vi "App - analyze RUS V6.vi"() -> ()   [LabVIEW 2015] (continued)
"radius"=0.0}}, "timestamp(min)"=1864.0666666701436, "timestamp"=timestamp(3493839665 s since 1904-01-01), "Magn Field(T)"=0.0}, {"temperature"=23.436, "lorentzian"={"Amplitude"=0.0, "omega(0)"=0.0, "Gamma"=0.0, "phase"=0.0, "Q"=0.0, "Norm  Ampl"=0.0, "z (inf)"=0.0+0.0i, "4corners"={"z (-pi/2)"=0.0+0.0i, "z(inf)"=0.0+0.0i, "z (pi/2)"=0.0+0.0i, "z center"=0.0+0.0i, "z(0)"=0.0+0.0i, "radius"=0.0}}, "timestamp(min)"=1865.3833333328366, "timestamp"=timestamp(3493839744 s since 1904-01-01), "Magn Field(T)"=0.0}, {"temperature"=23.334, "lorentzian"={"Amplitude"=0.0, "omega(0)"=0.0, "Gamma"=0.0, "phase"=0.0, "Q"=0.0, "Norm  Ampl"=0.0, "z (inf)"=0.0+0.0i, "4corners"={"z (-pi/2)"=0.0+0.0i, "z(inf)"=0.0+0.0i, "z (pi/2)"=0.0+0.0i, "z center"=0.0+0.0i, "z(0)"=0.0+0.0i, "radius"=0.0}}, "timestamp(min)"=1866.7000000029802, "timestamp"=timestamp(3493839823 s since 1904-01-01), "Magn Field(T)"=0.0}, {"temperature"=23.235, "lorentzian"={"Amplitude"=0.0, "omega(0)"=0.0, "Gamma"=0.0, "phase"=0.0, "Q"=0.0, "Norm  Ampl"=0.0, "z (inf)"=0.0+0.0i, "4corners"={"z (-pi/2)"=0.0+0.0i, "z(inf)"=0.0+0.0i, "z (pi/2)"=0.0+0.0i, "z center"=0.0+0.0i, "z(0)"=0.0+0.0i, "radius"=0.0}}, "timestamp(min)"=1868.0333333313465, "timestamp"=timestamp(3493839903 s since 1904-01-01), "Magn Field(T)"=0.0}, {"temperature"=23.139, "lorentzian"={"Amplitude"=0.0, "omega(0)"=0.0, "Gamma"=0.0, "phase"=0.0, "Q"=0.0, "Norm  Ampl"=0.0, "z (inf)"=0.0+0.0i, "4corners"={"z (-pi/2)"=0.0+0.0i, "z(inf)"=0.0+0.0i, "z (pi/2)"=0.0+0.0i, "z center"=0.0+0.0i, "z(0)"=0.0+0.0i, "radius"=0.0}}, "timestamp(min)"=1869.3500000014901, "timestamp"=timestamp(3493839982 s since 1904-01-01), "Magn Field(T)"=0.0}, {"temperature"=23.041, "lorentzian"={"Amplitude"=0.0, "omega(0)"=0.0, "Gamma"=0.0, "phase"=0.0, "Q"=0.0, "Norm  Ampl"=0.0, "z (inf)"=0.0+0.0i, "4corners"={"z (-pi/2)"=0.0+0.0i, "z(inf)"=0.0+0.0i, "z (pi/2)"=0.0+0.0i, "z center"=0.0+0.0i, "z(0)"=0.0+0.0i, "radius"=0.0}}, "timestamp(min)"=1870.683333337307, "timestamp"=timestamp(3493840062 s since 1904-01-01), "Magn Field(T)"=0.0}, {"temperature"=22.937, "lorentzian"={"Amplitude"=0.0, "omega(0)"=0.0, "Gamma"=0.0, "phase"=0.0, "Q"=0.0, "Norm  Ampl"=0.0, "z (inf)"=0.0+0.0i, "4corners"={"z (-pi/2)"=0.0+0.0i, "z(inf)"=0.0+0.0i, "z (pi/2)"=0.0+0.0i, "z center"=0.0+0.0i, "z(0)"=0.0+0.0i, "radius"=0.0}}, "timestamp(min)"=1872.0, "timestamp"=timestamp(3493840141 s since 1904-01-01), "Magn Field(T)"=0.0}, {"temperature"=22.842, "lorentzian"={"Amplitude"=0.0, "omega(0)"=0.0, "Gamma"=0.0, "phase"=0.0, "Q"=0.0, "Norm  Ampl"=0.0, "z (inf)"=0.0+0.0i, "4corners"={"z (-pi/2)"=0.0+0.0i, "z(inf)"=0.0+0.0i, "z (pi/2)"=0.0+0.0i, "z center"=0.0+0.0i, "z(0)"=0.0+0.0i, "radius"=0.0}}, "timestamp(min)"=1873.3166666701436, "timestamp"=timestamp(3493840220 s since 1904-01-01), "Magn Field(T)"=0.0}, {"temperature"=22.748, "lorentzian"={"Amplitude"=0.0, "omega(0)"=0.0, "Gamma"=0.0, "phase"=0.0, "Q"=0.0, "Norm  Ampl"=0.0, "z (inf)"=0.0+0.0i, "4corners"={"z (-pi/2)"=0.0+0.0i, "z(inf)"=0.0+0.0i, "z (pi/2)"=0.0+0.0i, "z center"=0.0+0.0i, "z(0)"=0.0+0.0i, "radius"=0.0}}, "timestamp(min)"=1874.6499999985099, "timestamp"=timestamp(3493840300 s since 1904-01-01), "Magn Field(T)"=0.0}, {"temperature"=22.644, "lorentzian"={"Amplitude"=0.0, "omega(0)"=0.0, "Gamma"=0.0, "phase"=0.0, "Q"=0.0, "Norm  Ampl"=0.0, "z (inf)"=0.0+0.0i, "4corners"={"z (-pi/2)"=0.0+0.0i, "z(inf)"=0.0+0.0i, "z (pi/2)"=0.0+0.0i, "z center"=0.0+0.0i, "z(0)"=0.0+0.0i, "radius"=0.0}}, "timestamp(min)"=1875.9666666686535, "timestamp"=timestamp(3493840379 s since 1904-01-01), "Magn Field(T)"=0.0}, {"temperature"=22.549, "lorentzian"={"Amplitude"=0.0, "omega(0)"=0.0, "Gamma"=0.0, "phase"=0.0, "Q"=0.0, "Norm  Ampl"=0.0, "z (inf)"=0.0+0.0i, "4corners"={"z (-pi/2)"=0.0+0.0i, "z(inf)"=0.0+0.0i, "z (pi/2)"=0.0+0.0i, "z center"=0.0+0.0i, "z(0)"=0.0+0.0i, "radius"=0.0}}, "timestamp(min)"=1877.2833333313465, "timestamp"=timestamp(3493840458 s since 1904-01-01), "Magn Field(T)"=0.0}, {"temperature"=22.448, "lorentzian"={"Amplitude"=0.0, "omega(0)"=0.0, "Gamma"=0.0, "phase"=0.0, "Q"=0.0, "Norm  Ampl"=0.0, "z (inf)"=0.0+0.0i, "4corners"={"z (-pi/2)"=0.0+0.0i, "z(inf)"=0.0+0.0i, "z (pi/2)"=0.0+0.0i, "z center"=0.0+0.0i, "z(0)"=0.0+0.0i, "radius"=0.0}}, "timestamp(min)"=1878.6166666671634, "timestamp"=timestamp(3493840538 s since 1904-01-01), "Magn Field(T)"=0.0}, {"temperature"=22.345, "lorentzian"={"Amplitude"=0.0, "omega(0)"=0.0, "Gamma"=0.0, "phase"=0.0, "Q"=0.0, "Norm  Ampl"=0.0, "z (inf)"=0.0+0.0i, "4corners"={"z (-pi/2)"=0.0+0.0i, "z(inf)"=0.0+0.0i, "z (pi/2)"=0.0+0.0i, "z center"=0.0+0.0i, "z(0)"=0.0+0.0i, "radius"=0.0}}, "timestamp(min)"=1879.933333337307, "timestamp"=timestamp(3493840617 s since 1904-01-01), "Magn Field(T)"=0.0}, {"temperature"=22.254, "lorentzian"={"Amplitude"=0.0, "omega(0)"=0.0, "Gamma"=0.0, "phase"=0.0, "Q"=0.0, "Norm  Ampl"=0.0, "z (inf)"=0.0+0.0i, "4corners"={"z (-pi/2)"=0.0+0.0i, "z(inf)"=0.0+0.0i, "z (pi/2)"=0.0+0.0i, "z center"=0.0+0.0i, "z(0)"=0.0+0.0i, "radius"=0.0}}, "timestamp(min)"=1881.2666666656733, "timestamp"=timestamp(3493840697 s since 1904-01-01), "Magn Field(T)"=0.0}, {"temperature"=22.148, "lorentzian"={"Amplitude"=0.0, "omega(0)"=0.0, "Gamma"=0.0, "phase"=0.0, "Q"=0.0, "Norm  Ampl"=0.0, "z (inf)"=0.0+0.0i, "4corners"={"z (-pi/2)"=0.0+0.0i, "z(inf)"=0.0+0.0i, "z (pi/2)"=0.0+0.0i, "z center"=0.0+0.0i, "z(0)"=0.0+0.0i, "radius"=0.0}}, "timestamp(min)"=1882.5833333358169, "timestamp"=timestamp(3493840776 s since 1904-01-01), "Magn Field(T)"=0.0}, {"temperature"=22.046, "lorentzian"={"Amplitude"=0.0, "omega(0)"=0.0, "Gamma"=0.0, "phase"=0.0, "Q"=0.0, "Norm  Ampl"=0.0, "z (inf)"=0.0+0.0i, "4corners"={"z (-pi/2)"=0.0+0.0i, "z(inf)"=0.0+0.0i, "z (pi/2)"=0.0+0.0i, "z center"=0.0+0.0i, "z(0)"=0.0+0.0i, "radius"=0.0}}, "timestamp(min)"=1883.8999999985099, "timestamp"=timestamp(3493840855 s since 1904-01-01), "Magn Field(T)"=0.0}, {"temperature"=21.957, "lorentzian"={"Amplitude"=0.0, "omega(0)"=0.0, "Gamma"=0.0, "phase"=0.0, "Q"=0.0, "Norm  Ampl"=0.0, "z (inf)"=0.0+0.0i, "4corners"={"z (-pi/2)"=0.0+0.0i, "z(inf)"=0.0+0.0i, "z (pi/2)"=0.0+0.0i, "z center"=0.0+0.0i, "z(0)"=0.0+0.0i, "radius"=0.0}}, "timestamp(min)"=1885.2333333343267, "timestamp"=timestamp(3493840935 s since 1904-01-01), "Magn Field(T)"=0.0}, {"temperature"=21.851, "lorentzian"={"Amplitude"=0.0, "omega(0)"=0.0, "Gamma"=0.0, "phase"=0.0, "Q"=0.0, "Norm  Ampl"=0.0, "z (inf)"=0.0+0.0i, "4corners"={"z (-pi/2)"=0.0+0.0i, "z(inf)"=0.0+0.0i, "z (pi/2)"=0.0+0.0i, "z center"=0.0+0.0i, "z(0)"=0.0+0.0i, "radius"=0.0}}, "timestamp(min)"=1886.5500000044703, "timestamp"=timestamp(3493841014 s since 1904-01-01), "Magn Field(T)"=0.0}, {"temperature"=21.755, "lorentzian"={"Amplitude"=0.0, "omega(0)"=0.0, "Gamma"=0.0, "phase"=0.0, "Q"=0.0, "Norm  Ampl"=0.0, "z (inf)"=0.0+0.0i, "4corners"={"z (-pi/2)"=0.0+0.0i, "z(inf)"=0.0+0.0i, "z (pi/2)"=0.0+0.0i, "z center"=0.0+0.0i, "z(0)"=0.0+0.0i, "radius"=0.0}}, "timestamp(min)"=1887.8833333328366, "timestamp"=timestamp(3493841094 s since 1904-01-01), "Magn Field(T)"=0.0}, {"temperature"=21.657, "lorentzian"={"Amplitude"=0.0, "omega(0)"=0.0, "Gamma"=0.0, "phase"=0.0, "Q"=0.0, "Norm  Ampl"=0.0, "z (inf)"=0.0+0.0i, "4corners"={"z (-pi/2)"=0.0+0.0i, "z(inf)"=0.0+0.0i, "z (pi/2)"=0.0+0.0i, "z center"=0.0+0.0i, "z(0)"=0.0+0.0i, "radius"=0.0}}, "timestamp(min)"=1889.2000000029802, "timestamp"=timestamp(3493841173 s since 1904-01-01), "Magn Field(T)"=0.0}, {"temperature"=21.553, "lorentzian"={"Amplitude"=0.0, "omega(0)"=0.0, "Gamma"=0.0, "phase"=0.0, "Q"=0.0, "Norm  Ampl"=0.0, "z (inf)"=0.0+0.0i, "4corners"={"z (-pi/2)"=0.0+0.0i, "z(inf)"=0.0+0.0i, "z (pi/2)"=0.0+0.0i, "z center"=0.0+0.0i, "z(0)"=0.0+0.0i, "radius"=0.0}}, "timestamp(min)"=1890.5166666656733, "timestamp"=timestamp(3493841252 s since 1904-01-01), "Magn Field(T)"=0.0}, {"temperature"=21.455, "lorentzian"={"Amplitude"=0.0, "omega(0)"=0.0, "Gamma"=0.0, "phase"=0.0, "Q"=0.0, "Norm  Ampl"=0.0, "z (inf)"=0.0+0.0i, "4corners"={"z (-pi/2)"=0.0+0.0i, "z(inf)"=0.0+0.0i, "z (pi/2)"=0.0+0.0i, "z center"=0.0+0.0i, "z(0)"=0.0+0.0i, "radius"=0.0}}, "timestamp(min)"=1891.8500000014901, "timestamp"=timestamp(3493841332 s since 1904-01-01), "Magn Field(T)"=0.0}, {"temperature"=21.36, "lorentzian"={"Amplitude"=0.0, "omega(0)"=0.0, "Gamma"=0.0, "phase"=0.0, "Q"=0.0, "Norm  Ampl"=0.0, "z (inf)"=0.0+0.0i, "4corners"={"z (-pi/2)"=0.0+0.0i, "z(inf)"=0.0+0.0i, "z (pi/2)"=0.0+0.0i, "z center"=0.0+0.0i, "z(0)"=0.0+0.0i, "radius"=0.0}}, "timestamp(min)"=1893.1666666641831, "timestamp"=timestamp(3493841411 s since 1904-01-01), "Magn Field(T)"=0.0}, {"temperature"=21.259, "lorentzian"={"Amplitude"=0.0, "omega(0)"=0.0, "Gamma"=0.0, "phase"=0.0, "Q"=0.0, "Norm  Ampl"=0.0, "z (inf)"=0.0+0.0i, "4corners"={"z (-pi/2)"=0.0+0.0i, "z(inf)"=0.0+0.0i, "z (pi/2)"=0.0+0.0i, "z center"=0.0+0.0i, "z(0)"=0.0+0.0i, "radius"=0.0}}, "timestamp(min)"=1894.4833333343267, "timestamp"=timestamp(3493841490 s since 1904-01-01), "Magn Field(T)"=0.0}, {"temperature"=21.158, "lorentzian"={"Amplitude"=0.0, "omega(0)"=0.0, "Gamma"=0.0, "phase"=0.0, "Q"=0.0, "Norm  Ampl"=0.0, "z (inf)"=0.0+0.0i, "4corners"={"z (-pi/2)"=0.0+0.0i, "z(inf)"=0.0+0.0i, "z (pi/2)"=0.0+0.0i, "z center"=0.0+0.0i, "z(0)"=0.0+0.0i, "radius"=0.0}}, "timestamp(min)"=1895.8166666701436, "timestamp"=timestamp(3493841570 s since 1904-01-01), "Magn Field(T)"=0.0}, {"temperature"=21.06, "lorentzian"={"Amplitude"=0.0, "omega(0)"=0.0, "Gamma"=0.0, "phase"=0.0, "Q"=0.0, "Norm  Ampl"=0.0, "z (inf)"=0.0+0.0i, "4corners"={"z (-pi/2)"=0.0+0.0i, "z(inf)"=0.0+0.0i, "z (pi/2)"=0.0+0.0i, "z center"=0.0+0.0i, "z(0)"=0.0+0.0i, "radius"=0.0}}, "timestamp(min)"=1897.1333333328366, "timestamp"=timestamp(3493841649 s since 1904-01-01), "Magn Field(T)"=0.0}, {"temperature"=20.959, "lorentzian"={"Amplitude"=0.0, "omega(0)"=0.0, "Gamma"=0.0, "phase"=0.0, "Q"=0.0, "Norm  Ampl"=0.0, "z (inf)"=0.0+0.0i, "4corners"={"z (-pi/2)"=0.0+0.0i, "z(inf)"=0.0+0.0i, "z (pi/2)"=0.0+0.0i, "z center"=0.0+0.0i, "z(0)"=0.0+0.0i, "radius"=0.0}}, "timestamp(min)"=1898.4666666686535, "timestamp"=timestamp(3493841729 s since 1904-01-01), "Magn Field(T)"=0.0}, {"temperature"=20.861, "lorentzian"={"Amplitude"=0.0, "omega(0)"=0.0, "Gamma"=0.0, "phase"=0.0, "Q"=0.0, "Norm  Ampl"=0.0, "z (inf)"=0.0+0.0i, "4corners"={"z (-pi/2)"=0.0+0.0i, "z(inf)"=0.0+0.0i, "z (pi/2)"=0.0+0.0i, "z center"=0.0+0.0i, "z(0)"=0.0+0.0i, "radius"=0.0}}, "timestamp(min)"=1899.7833333313465, "timestamp"=timestamp(3493841808 s since 1904-01-01), "Magn Field(T)"=0.0}, {"temperature"=20.758, "lorentzian"={"Amplitude"=0.0, "omega(0)"=0.0, "Gamma"=0.0, "phase"=0.0, "Q"=0.0, "Norm  Ampl"=0.0, "z (inf)"=0.0+0.0i, "4corners"={"z (-pi/2)"=0.0+0.0i, "z(inf)"=0.0+0.0i, "z (pi/2)"=0.0+0.0i, "z center"=0.0+0.0i, "z(0)"=0.0+0.0i, "radius"=0.0}}, "timestamp(min)"=1901.1000000014901, "timestamp"=timestamp(3493841887 s since 1904-01-01), "Magn Field(T)"=0.0}, {"temperature"=20.654, "lorentzian"={"Amplitude"=0.0, "omega(0)"=0.0, "Gamma"=0.0, "phase"=0.0, "Q"=0.0, "Norm  Ampl"=0.0, "z (inf)"=0.0+0.0i, "4corners"={"z (-pi/2)"=0.0+0.0i, "z(inf)"=0.0+0.0i, "z (pi/2)"=0.0+0.0i, "z center"=0.0+0.0i, "z(0)"=0.0+0.0i, "radius"=0.0}}, "timestamp(min)"=1902.433333337307, "timestamp"=timestamp(3493841967 s since 1904-01-01), "Magn Field(T)"=0.0}, {"temperature"=20.555, "lorentzian"={"Amplitude"=0.0, "omega(0)"=0.0, "Gamma"=0.0, "phase"=0.0, "Q"=0.0, "Norm  Ampl"=0.0, "z (inf)"=0.0+0.0i, "4corners"={"z (-pi/2)"=0.0+0.0i, "z(inf)"=0.0+0.0i, "z (pi/2)"=0.0+0.0i, "z center"=0.0+0.0i, "z(0)"=0.0+0.0i, "radius"=0.0}}, "timestamp(min)"=1903.75, "timestamp"=timestamp(3493842046 s since 1904-01-01), "Magn Field(T)"=0.0}, {"temperature"=20.461, "lorentzian"={"Amplitude"=0.0, "omega(0)"=0.0, "Gamma"=0.0, "phase"=0.0, "Q"=0.0, "Norm  Ampl"=0.0, "z (inf)"=0.0+0.0i, "4corners"={"z (-pi/2)"=0.0+0.0i, "z(inf)"=0.0+0.0i, "z (pi/2)"=0.0+0.0i, "z center"=0.0+0.0i, "z(0)"=0.0+0.0i, "radius"=0.0}}, "timestamp(min)"=1905.0666666701436, "timestamp"=timestamp(3493842125 s since 1904-01-01), "Magn Field(T)"=0.0}, {"temperature"=20.355, "lorentzian"={"Amplitude"=0.0, "omega(0)"=0.0, "Gamma"=0.0, "phase"=0.0, "Q"=0.0, "Norm  Ampl"=0.0, "z (inf)"=0.0+0.0i, "4corners"={"z (-pi/2)"=0.0+0.0i, "z(inf)"=0.0+0.0i, "z (pi/2)"=0.0+0.0i, "z center"=0.0+0.0i, "z(0)"=0.0+0.0i, "radius"=0.0}}, "timestamp(min)"=1906.3999999985099, "timestamp"=timestamp(3493842205 s since 1904-01-01), "Magn Field(T)"=0.0}, {"temperature"=20.262, "lorentzian"={"Amplitude"=0.0, "omega(0)"=0.0, "Gamma"=0.0, "phase"=0.0, "Q"=0.0, "Norm  Ampl"=0.0, "z (inf)"=0.0+0.0i, "4corners"={"z (-pi/2)"=0.0+0.0i, "z(inf)"=0.0+0.0i, "z (pi/2)"=0.0+0.0i, "z center"=0.0+0.0i, "z(0)"=0.0+0.0i, "radius"=0.0}}, "timestamp(min)"=1907.7166666686535, "timestamp"=timestamp(3493842284 s since 1904-01-01), "Magn Field(T)"=0.0}, {"temperature"=20.157, "lorentzian"={"Amplitude"=0.0, "omega(0)"=0.0, "Gamma"=0.0, "phase"=0.0, "Q"=0.0, "Norm  Ampl"=0.0, "z (inf)"=0.0+0.0i, "4corners"={"z (-pi/2)"=0.0+0.0i, "z(inf)"=0.0+0.0i, "z (pi/2)"=0.0+0.0i, "z center"=0.0+0.0i, "z(0)"=0.0+0.0i, "radius"=0.0}}, "timestamp(min)"=1909.0500000044703, "timestamp"=timestamp(3493842364 s since 1904-01-01), "Magn Field(T)"=0.0}, {"temperature"=20.054, "lorentzian"={"Amplitude"=0.0, "omega(0)"=0.0, "Gamma"=0.0, "phase"=0.0, "Q"=0.0, "Norm  Ampl"=0.0, "z (inf)"=0.0+0.0i, "4corners"={"z (-pi/2)"=0.0+0.0i, "z(inf)"=0.0+0.0i, "z (pi/2)"=0.0+0.0i, "z center"=0.0+0.0i, "z(0)"=0.0+0.0i, "radius"=0.0}}, "timestamp(min)"=1910.3666666671634, "timestamp"=timestamp(3493842443 s since 1904-01-01), "Magn Field(T)"=0.0}, {"temperature"=19.964, "lorentzian"={"Amplitude"=0.0, "omega(0)"=0.0, "Gamma"=0.0, "phase"=0.0, "Q"=0.0, "Norm  Ampl"=0.0, "z (inf)"=0.0+0.0i, "4corners"={"z (-pi/2)"=0.0+0.0i, "z(inf)"=0.0+0.0i, "z (pi/2)"=0.0+0.0i, "z center"=0.0+0.0i, "z(0)"=0.0+0.0i, "radius"=0.0}}, "timestamp(min)"=1911.683333337307, "timestamp"=timestamp(3493842522 s since 1904-01-01), "Magn Field(T)"=0.0}, {"temperature"=19.857, "lorentzian"={"Amplitude"=0.0, "omega(0)"=0.0, "Gamma"=0.0, "phase"=0.0, "Q"=0.0, "Norm  Ampl"=0.0, "z (inf)"=0.0+0.0i, "4corners"={"z (-pi/2)"=0.0+0.0i, "z(inf)"=0.0+0.0i, "z (pi/2)"=0.0+0.0i, "z center"=0.0+0.0i, "z(0)"=0.0+0.0i, "radius"=0.0}}, "timestamp(min)"=1913.0166666656733, "timestamp"=timestamp(3493842602 s since 1904-01-01), "Magn Field(T)"=0.0}, {"temperature"=19.754, "lorentzian"={"Amplitude"=0.0, "omega(0)"=0.0, "Gamma"=0.0, "phase"=0.0, "Q"=0.0, "Norm  Ampl"=0.0, "z (inf)"=0.0+0.0i, "4corners"={"z (-pi/2)"=0.0+0.0i, "z(inf)"=0.0+0.0i, "z (pi/2)"=0.0+0.0i, "z center"=0.0+0.0i, "z(0)"=0.0+0.0i, "radius"=0.0}}, "timestamp(min)"=1914.3333333358169, "timestamp"=timestamp(3493842681 s since 1904-01-01), "Magn Field(T)"=0.0}, {"temperature"=19.658, "lorentzian"={"Amplitude"=0.0, "omega(0)"=0.0, "Gamma"=0.0, "phase"=0.0, "Q"=0.0, "Norm  Ampl"=0.0, "z (inf)"=0.0+0.0i, "4corners"={"z (-pi/2)"=0.0+0.0i, "z(inf)"=0.0+0.0i, "z (pi/2)"=0.0+0.0i, "z center"=0.0+0.0i, "z(0)"=0.0+0.0i, "radius"=0.0}}, "timestamp(min)"=1915.6666666641831, "timestamp"=timestamp(3493842761 s since 1904-01-01), "Magn Field(T)"=0.0}, {"temperature"=19.556, "lorentzian"={"Amplitude"=0.0, "omega(0)"=0.0, "Gamma"=0.0, "phase"=0.0, "Q"=0.0, "Norm  Ampl"=0.0, "z (inf)"=0.0+0.0i, "4corners"={"z (-pi/2)"=0.0+0.0i, "z(inf)"=0.0+0.0i, "z (pi/2)"=0.0+0.0i, "z center"=0.0+0.0i, "z(0)"=0.0+0.0i, "radius"=0.0}}, "timestamp(min)"=1916.9833333343267, "timestamp"=timestamp(3493842840 s since 1904-01-01), "Magn Field(T)"=0.0}, {"temperature"=19.452, "lorentzian"={"Amplitude"=0.0, "omega(0)"=0.0, "Gamma"=0.0, "phase"=0.0, "Q"=0.0, "Norm  Ampl"=0.0, "z (inf)"=0.0+0.0i, "4corners"={"z (-pi/2)"=0.0+0.0i, "z(inf)"=0.0+0.0i, "z (pi/2)"=0.0+0.0i, "z center"=0.0+0.0i, "z(0)"=0.0+0.0i, "radius"=0.0}}, "timestamp(min)"=1918.3000000044703, "timestamp"=timestamp(3493842919 s since 1904-01-01), "Magn Field(T)"=0.0}, {"temperature"=19.356, "lorentzian"={"Amplitude"=0.0, "omega(0)"=0.0, "Gamma"=0.0, "phase"=0.0, "Q"=0.0, "Norm  Ampl"=0.0, "z (inf)"=0.0+0.0i, "4corners"={"z (-pi/2)"=0.0+0.0i, "z(inf)"=0.0+0.0i, "z (pi/2)"=0.0+0.0i, "z center"=0.0+0.0i, "z(0)"=0.0+0.0i, "radius"=0.0}}, "timestamp(min)"=1919.6333333328366, "timestamp"=timestamp(3493842999 s since 1904-01-01), "Magn Field(T)"=0.0}, {"temperature"=19.258, "lorentzian"={"Amplitude"=0.0, "omega(0)"=0.0, "Gamma"=0.0, "phase"=0.0, "Q"=0.0, "Norm  Ampl"=0.0, "z (inf)"=0.0+0.0i, "4corners"={"z (-pi/2)"=0.0+0.0i, "z(inf)"=0.0+0.0i, "z (pi/2)"=0.0+0.0i, "z center"=0.0+0.0i, "z(0)"=0.0+0.0i, "radius"=0.0}}, "timestamp(min)"=1920.9500000029802, "timestamp"=timestamp(3493843078 s since 1904-01-01), "Magn Field(T)"=0.0}, {"temperature"=19.154, "lorentzian"={"Amplitude"=0.0, "omega(0)"=0.0, "Gamma"=0.0, "phase"=0.0, "Q"=0.0, "Norm  Ampl"=0.0, "z (inf)"=0.0+0.0i, "4corners"={"z (-pi/2)"=0.0+0.0i, "z(inf)"=0.0+0.0i, "z (pi/2)"=0.0+0.0i, "z center"=0.0+0.0i, "z(0)"=0.0+0.0i, "radius"=0.0}}, "timestamp(min)"=1922.2666666656733, "timestamp"=timestamp(3493843157 s since 1904-01-01), "Magn Field(T)"=0.0}, {"temperature"=19.054, "lorentzian"={"Amplitude"=0.0, "omega(0)"=0.0, "Gamma"=0.0, "phase"=0.0, "Q"=0.0, "Norm  Ampl"=0.0, "z (inf)"=0.0+0.0i, "4corners"={"z (-pi/2)"=0.0+0.0i, "z(inf)"=0.0+0.0i, "z (pi/2)"=0.0+0.0i, "z center"=0.0+0.0i, "z(0)"=0.0+0.0i, "radius"=0.0}}, "timestamp(min)"=1923.6000000014901, "timestamp"=timestamp(3493843237 s since 1904-01-01), "Magn Field(T)"=0.0}, {"temperature"=18.951, "lorentzian"={"Amplitude"=0.0, "omega(0)"=0.0, "Gamma"=0.0, "phase"=0.0, "Q"=0.0, "Norm  Ampl"=0.0, "z (inf)"=0.0+0.0i, "4corners"={"z (-pi/2)"=0.0+0.0i, "z(inf)"=0.0+0.0i, "z (pi/2)"=0.0+0.0i, "z center"=0.0+0.0i, "z(0)"=0.0+0.0i, "radius"=0.0}}, "timestamp(min)"=1924.9166666641831, "timestamp"=timestamp(3493843316 s since 1904-01-01), "Magn Field(T)"=0.0}, {"temperature"=18.852, "lorentzian"={"Amplitude"=0.0, "omega(0)"=0.0, "Gamma"=0.0, "phase"=0.0, "Q"=0.0, "Norm  Ampl"=0.0, "z (inf)"=0.0+0.0i, "4corners"={"z (-pi/2)"=0.0+0.0i, "z(inf)"=0.0+0.0i, "z (pi/2)"=0.0+0.0i, "z center"=0.0+0.0i, "z(0)"=0.0+0.0i, "radius"=0.0}}, "timestamp(min)"=1926.25, "timestamp"=timestamp(3493843396 s since 1904-01-01), "Magn Field(T)"=0.0}, {"temperature"=18.757, "lorentzian"={"Amplitude"=0.0, "omega(0)"=0.0, "Gamma"=0.0, "phase"=0.0, "Q"=0.0, "Norm  Ampl"=0.0, "z (inf)"=0.0+0.0i, "4corners"={"z (-pi/2)"=0.0+0.0i, "z(inf)"=0.0+0.0i, "z (pi/2)"=0.0+0.0i, "z center"=0.0+0.0i, "z(0)"=0.0+0.0i, "radius"=0.0}}, "timestamp(min)"=1927.5666666701436, "timestamp"=timestamp(3493843475 s since 1904-01-01), "Magn Field(T)"=0.0}, {"temperature"=18.649, "lorentzian"={"Amplitude"=0.0, "omega(0)"=0.0, "Gamma"=0.0, "phase"=0.0, "Q"=0.0, "Norm  Ampl"=0.0, "z (inf)"=0.0+0.0i, "4corners"={"z (-pi/2)"=0.0+0.0i, "z(inf)"=0.0+0.0i, "z (pi/2)"=0.0+0.0i, "z center"=0.0+0.0i, "z(0)"=0.0+0.0i, "radius"=0.0}}, "timestamp(min)"=1928.8833333328366, "timestamp"=timestamp(3493843554 s since 1904-01-01), "Magn Field(T)"=0.0}, {"temperature"=18.548, "lorentzian"={"Amplitude"=0.0, "omega(0)"=0.0, "Gamma"=0.0, "phase"=0.0, "Q"=0.0, "Norm  Ampl"=0.0, "z (inf)"=0.0+0.0i, "4corners"={"z (-pi/2)"=0.0+0.0i, "z(inf)"=0.0+0.0i, "z (pi/2)"=0.0+0.0i, "z center"=0.0+0.0i, "z(0)"=0.0+0.0i, "radius"=0.0}}, "timestamp(min)"=1930.2166666686535, "timestamp"=timestamp(3493843634 s since 1904-01-01), "Magn Field(T)"=0.0}, {"temperature"=18.451, "lorentzian"={"Amplitude"=0.0, "omega(0)"=0.0, "Gamma"=0.0, "phase"=0.0, "Q"=0.0, "Norm  Ampl"=0.0, "z (inf)"=0.0+0.0i, "4corners"={"z (-pi/2)"=0.0+0.0i, "z(inf)"=0.0+0.0i, "z (pi/2)"=0.0+0.0i, "z center"=0.0+0.0i, "z(0)"=0.0+0.0i, "radius"=0.0}}, "timestamp(min)"=1931.5333333313465, "timestamp"=timestamp(3493843713 s since 1904-01-01), "Magn Field(T)"=0.0}, {"temperature"=18.346, "lorentzian"={"Amplitude"=0.0, "omega(0)"=0.0, "Gamma"=0.0, "phase"=0.0, "Q"=0.0, "Norm  Ampl"=0.0, "z (inf)"=0.0+0.0i, "4corners"={"z (-pi/2)"=0.0+0.0i, "z(inf)"=0.0+0.0i, "z (pi/2)"=0.0+0.0i, "z center"=0.0+0.0i, "z(0)"=0.0+0.0i, "radius"=0.0}}, "timestamp(min)"=1932.8666666671634, "timestamp"=timestamp(3493843793 s since 1904-01-01), "Magn Field(T)"=0.0}, {"temperature"=18.245, "lorentzian"={"Amplitude"=0.0, "omega(0)"=0.0, "Gamma"=0.0, "phase"=0.0, "Q"=0.0, "Norm  Ampl"=0.0, "z (inf)"=0.0+0.0i, "4corners"={"z (-pi/2)"=0.0+0.0i, "z(inf)"=0.0+0.0i, "z (pi/2)"=0.0+0.0i, "z center"=0.0+0.0i, "z(0)"=0.0+0.0i, "radius"=0.0}}, "timestamp(min)"=1934.183333337307, "timestamp"=timestamp(3493843872 s since 1904-01-01), "Magn Field(T)"=0.0}, {"temperature"=18.147, "lorentzian"={"Amplitude"=0.0, "omega(0)"=0.0, "Gamma"=0.0, "phase"=0.0, "Q"=0.0, "Norm  Ampl"=0.0, "z (inf)"=0.0+0.0i, "4corners"={"z (-pi/2)"=0.0+0.0i, "z(inf)"=0.0+0.0i, "z (pi/2)"=0.0+0.0i, "z center"=0.0+0.0i, "z(0)"=0.0+0.0i, "radius"=0.0}}, "timestamp(min)"=1935.5, "timestamp"=timestamp(3493843951 s since 1904-01-01), "Magn Field(T)"=0.0}, {"temperature"=18.042, "lorentzian"={"Amplitude"=0.0, "omega(0)"=0.0, "Gamma"=0.0, "phase"=0.0, "Q"=0.0, "Norm  Ampl"=0.0, "z (inf)"=0.0+0.0i, "4corners"={"z (-pi/2)"=0.0+0.0i, "z(inf)"=0.0+0.0i, "z (pi/2)"=0.0+0.0i, "z center"=0.0+0.0i, "z(0)"=0.0+0.0i, "radius"=0.0}}, "timestamp(min)"=1936.8333333358169, "timestamp"=timestamp(3493844031 s since 1904-01-01), "Magn Field(T)"=0.0}, {"temperature"=17.951, "lorentzian"={"Amplitude"=0.0, "omega(0)"=0.0, "Gamma"=0.0, "phase"=0.0, "Q"=0.0, "Norm  Ampl"=0.0, "z (inf)"=0.0+0.0i, "4corners"={"z (-pi/2)"=0.0+0.0i, "z(inf)"=0.0+0.0i, "z (pi/2)"=0.0+0.0i, "z center"=0.0+0.0i, "z(0)"=0.0+0.0i, "radius"=0.0}}, "timestamp(min)"=1938.1499999985099, "timestamp"=timestamp(3493844110 s since 1904-01-01), "Magn Field(T)"=0.0}, {"temperature"=17.844, "lorentzian"={"Amplitude"=0.0, "omega(0)"=0.0, "Gamma"=0.0, "phase"=0.0, "Q"=0.0, "Norm  Ampl"=0.0, "z (inf)"=0.0+0.0i, "4corners"={"z (-pi/2)"=0.0+0.0i, "z(inf)"=0.0+0.0i, "z (pi/2)"=0.0+0.0i, "z center"=0.0+0.0i, "z(0)"=0.0+0.0i, "radius"=0.0}}, "timestamp(min)"=1939.4666666686535, "timestamp"=timestamp(3493844189 s since 1904-01-01), "Magn Field(T)"=0.0}, {"temperature"=17.735, "lorentzian"={"Amplitude"=0.0, "omega(0)"=0.0, "Gamma"=0.0, "phase"=0.0, "Q"=0.0, "Norm  Ampl"=0.0, "z (inf)"=0.0+0.0i, "4corners"={"z (-pi/2)"=0.0+0.0i, "z(inf)"=0.0+0.0i, "z (pi/2)"=0.0+0.0i, "z center"=0.0+0.0i, "z(0)"=0.0+0.0i, "radius"=0.0}}, "timestamp(min)"=1940.8000000044703, "timestamp"=timestamp(3493844269 s since 1904-01-01), "Magn Field(T)"=0.0}, {"temperature"=17.643, "lorentzian"={"Amplitude"=0.0, "omega(0)"=0.0, "Gamma"=0.0, "phase"=0.0, "Q"=0.0, "Norm  Ampl"=0.0, "z (inf)"=0.0+0.0i, "4corners"={"z (-pi/2)"=0.0+0.0i, "z(inf)"=0.0+0.0i, "z (pi/2)"=0.0+0.0i, "z center"=0.0+0.0i, "z(0)"=0.0+0.0i, "radius"=0.0}}, "timestamp(min)"=1942.1166666671634, "timestamp"=timestamp(3493844348 s since 1904-01-01), "Magn Field(T)"=0.0}, {"temperature"=17.54, "lorentzian"={"Amplitude"=0.0, "omega(0)"=0.0, "Gamma"=0.0, "phase"=0.0, "Q"=0.0, "Norm  Ampl"=0.0, "z (inf)"=0.0+0.0i, "4corners"={"z (-pi/2)"=0.0+0.0i, "z(inf)"=0.0+0.0i, "z (pi/2)"=0.0+0.0i, "z center"=0.0+0.0i, "z(0)"=0.0+0.0i, "radius"=0.0}}, "timestamp(min)"=1943.4500000029802, "timestamp"=timestamp(3493844428 s since 1904-01-01), "Magn Field(T)"=0.0}, {"temperature"=17.438, "lorentzian"={"Amplitude"=0.0, "omega(0)"=0.0, "Gamma"=0.0, "phase"=0.0, "Q"=0.0, "Norm  Ampl"=0.0, "z (inf)"=0.0+0.0i, "4corners"={"z (-pi/2)"=0.0+0.0i, "z(inf)"=0.0+0.0i, "z (pi/2)"=0.0+0.0i, "z center"=0.0+0.0i, "z(0)"=0.0+0.0i, "radius"=0.0}}, "timestamp(min)"=1944.7666666656733, "timestamp"=timestamp(3493844507 s since 1904-01-01), "Magn Field(T)"=0.0}, {"temperature"=17.338, "lorentzian"={"Amplitude"=0.0, "omega(0)"=0.0, "Gamma"=0.0, "phase"=0.0, "Q"=0.0, "Norm  Ampl"=0.0, "z (inf)"=0.0+0.0i, "4corners"={"z (-pi/2)"=0.0+0.0i, "z(inf)"=0.0+0.0i, "z (pi/2)"=0.0+0.0i, "z center"=0.0+0.0i, "z(0)"=0.0+0.0i, "radius"=0.0}}, "timestamp(min)"=1946.0833333358169, "timestamp"=timestamp(3493844586 s since 1904-01-01), "Magn Field(T)"=0.0}, {"temperature"=17.235, "lorentzian"={"Amplitude"=0.0, "omega(0)"=0.0, "Gamma"=0.0, "phase"=0.0, "Q"=0.0, "Norm  Ampl"=0.0, "z (inf)"=0.0+0.0i, "4corners"={"z (-pi/2)"=0.0+0.0i, "z(inf)"=0.0+0.0i, "z (pi/2)"=0.0+0.0i, "z center"=0.0+0.0i, "z(0)"=0.0+0.0i, "radius"=0.0}}, "timestamp(min)"=1947.4166666641831, "timestamp"=timestamp(3493844666 s since 1904-01-01), "Magn Field(T)"=0.0}, {"temperature"=17.133, "lorentzian"={"Amplitude"=0.0, "omega(0)"=0.0, "Gamma"=0.0, "phase"=0.0, "Q"=0.0, "Norm  Ampl"=0.0, "z (inf)"=0.0+0.0i, "4corners"={"z (-pi/2)"=0.0+0.0i, "z(inf)"=0.0+0.0i, "z (pi/2)"=0.0+0.0i, "z center"=0.0+0.0i, "z(0)"=0.0+0.0i, "radius"=0.0}}, "timestamp(min)"=1948.7333333343267, "timestamp"=timestamp(3493844745 s since 1904-01-01), "Magn Field(T)"=0.0}, {"temperature"=17.034, "lorentzian"={"Amplitude"=0.0, "omega(0)"=0.0, "Gamma"=0.0, "phase"=0.0, "Q"=0.0, "Norm  Ampl"=0.0, "z (inf)"=0.0+0.0i, "4corners"={"z (-pi/2)"=0.0+0.0i, "z(inf)"=0.0+0.0i, "z (pi/2)"=0.0+0.0i, "z center"=0.0+0.0i, "z(0)"=0.0+0.0i, "radius"=0.0}}, "timestamp(min)"=1950.0500000044703, "timestamp"=timestamp(3493844824 s since 1904-01-01), "Magn Field(T)"=0.0}, {"temperature"=16.936, "lorentzian"={"Amplitude"=0.0, "omega(0)"=0.0, "Gamma"=0.0, "phase"=0.0, "Q"=0.0, "Norm  Ampl"=0.0, "z (inf)"=0.0+0.0i, "4corners"={"z (-pi/2)"=0.0+0.0i, "z(inf)"=0.0+0.0i, "z (pi/2)"=0.0+0.0i, "z center"=0.0+0.0i, "z(0)"=0.0+0.0i, "radius"=0.0}}, "timestamp(min)"=1951.3833333328366, "timestamp"=timestamp(3493844904 s since 1904-01-01), "Magn Field(T)"=0.0}, {"temperature"=16.831, "lorentzian"={"Amplitude"=0.0, "omega(0)"=0.0, "Gamma"=0.0, "phase"=0.0, "Q"=0.0, "Norm  Ampl"=0.0, "z (inf)"=0.0+0.0i, "4corners"={"z (-pi/2)"=0.0+0.0i, "z(inf)"=0.0+0.0i, "z (pi/2)"=0.0+0.0i, "z center"=0.0+0.0i, "z(0)"=0.0+0.0i, "radius"=0.0}}, "timestamp(min)"=1952.7000000029802, "timestamp"=timestamp(3493844983 s since 1904-01-01), "Magn Field(T)"=0.0}, {"temperature"=16.732, "lorentzian"={"Amplitude"=0.0, "omega(0)"=0.0, "Gamma"=0.0, "phase"=0.0, "Q"=0.0, "Norm  Ampl"=0.0, "z (inf)"=0.0+0.0i, "4corners"={"z (-pi/2)"=0.0+0.0i, "z(inf)"=0.0+0.0i, "z (pi/2)"=0.0+0.0i, "z center"=0.0+0.0i, "z(0)"=0.0+0.0i, "radius"=0.0}}, "timestamp(min)"=1954.0333333313465, "timestamp"=timestamp(3493845063 s since 1904-01-01), "Magn Field(T)"=0.0}, {"temperature"=16.631, "lorentzian"={"Amplitude"=0.0, "omega(0)"=0.0, "Gamma"=0.0, "phase"=0.0, "Q"=0.0, "Norm  Ampl"=0.0, "z (inf)"=0.0+0.0i, "4corners"={"z (-pi/2)"=0.0+0.0i, "z(inf)"=0.0+0.0i, "z (pi/2)"=0.0+0.0i, "z center"=0.0+0.0i, "z(0)"=0.0+0.0i, "radius"=0.0}}, "timestamp(min)"=1955.3500000014901, "timestamp"=timestamp(3493845142 s since 1904-01-01), "Magn Field(T)"=0.0}, {"temperature"=16.524, "lorentzian"={"Amplitude"=0.0, "omega(0)"=0.0, "Gamma"=0.0, "phase"=0.0, "Q"=0.0, "Norm  Ampl"=0.0, "z (inf)"=0.0+0.0i, "4corners"={"z (-pi/2)"=0.0+0.0i, "z(inf)"=0.0+0.0i, "z (pi/2)"=0.0+0.0i, "z center"=0.0+0.0i, "z(0)"=0.0+0.0i, "radius"=0.0}}, "timestamp(min)"=1956.6666666641831, "timestamp"=timestamp(3493845221 s since 1904-01-01), "Magn Field(T)"=0.0}, {"temperature"=16.433, "lorentzian"={"Amplitude"=0.0, "omega(0)"=0.0, "Gamma"=0.0, "phase"=0.0, "Q"=0.0, "Norm  Ampl"=0.0, "z (inf)"=0.0+0.0i, "4corners"={"z (-pi/2)"=0.0+0.0i, "z(inf)"=0.0+0.0i, "z (pi/2)"=0.0+0.0i, "z center"=0.0+0.0i, "z(0)"=0.0+0.0i, "radius"=0.0}}, "timestamp(min)"=1958.0, "timestamp"=timestamp(3493845301 s since 1904-01-01), "Magn Field(T)"=0.0}, {"temperature"=16.322, "lorentzian"={"Amplitude"=0.0, "omega(0)"=0.0, "Gamma"=0.0, "phase"=0.0, "Q"=0.0, "Norm  Ampl"=0.0, "z (inf)"=0.0+0.0i, "4corners"={"z (-pi/2)"=0.0+0.0i, "z(inf)"=0.0+0.0i, "z (pi/2)"=0.0+0.0i, "z center"=0.0+0.0i, "z(0)"=0.0+0.0i, "radius"=0.0}}, "timestamp(min)"=1959.3166666701436, "timestamp"=timestamp(3493845380 s since 1904-01-01), "Magn Field(T)"=0.0}, {"temperature"=16.223, "lorentzian"={"Amplitude"=0.0, "omega(0)"=0.0, "Gamma"=0.0, "phase"=0.0, "Q"=0.0, "Norm  Ampl"=0.0, "z (inf)"=0.0+0.0i, "4corners"={"z (-pi/2)"=0.0+0.0i, "z(inf)"=0.0+0.0i, "z (pi/2)"=0.0+0.0i, "z center"=0.0+0.0i, "z(0)"=0.0+0.0i, "radius"=0.0}}, "timestamp(min)"=1960.6499999985099, "timestamp"=timestamp(3493845460 s since 1904-01-01), "Magn Field(T)"=0.0}, {"temperature"=16.128, "lorentzian"={"Amplitude"=0.0, "omega(0)"=0.0, "Gamma"=0.0, "phase"=0.0, "Q"=0.0, "Norm  Ampl"=0.0, "z (inf)"=0.0+0.0i, "4corners"={"z (-pi/2)"=0.0+0.0i, "z(inf)"=0.0+0.0i, "z (pi/2)"=0.0+0.0i, "z center"=0.0+0.0i, "z(0)"=0.0+0.0i, "radius"=0.0}}, "timestamp(min)"=1961.9666666686535, "timestamp"=timestamp(3493845539 s since 1904-01-01), "Magn Field(T)"=0.0}, {"temperature"=16.024, "lorentzian"={"Amplitude"=0.0, "omega(0)"=0.0, "Gamma"=0.0, "phase"=0.0, "Q"=0.0, "Norm  Ampl"=0.0, "z (inf)"=0.0+0.0i, "4corners"={"z (-pi/2)"=0.0+0.0i, "z(inf)"=0.0+0.0i, "z (pi/2)"=0.0+0.0i, "z center"=0.0+0.0i, "z(0)"=0.0+0.0i, "radius"=0.0}}, "timestamp(min)"=1963.2833333313465, "timestamp"=timestamp(3493845618 s since 1904-01-01), "Magn Field(T)"=0.0}, {"temperature"=15.924, "lorentzian"={"Amplitude"=0.0, "omega(0)"=0.0, "Gamma"=0.0, "phase"=0.0, "Q"=0.0, "Norm  Ampl"=0.0, "z (inf)"=0.0+0.0i, "4corners"={"z (-pi/2)"=0.0+0.0i, "z(inf)"=0.0+0.0i, "z (pi/2)"=0.0+0.0i, "z center"=0.0+0.0i, "z(0)"=0.0+0.0i, "radius"=0.0}}, "timestamp(min)"=1964.6166666671634, "timestamp"=timestamp(3493845698 s since 1904-01-01), "Magn Field(T)"=0.0}, {"temperature"=15.82, "lorentzian"={"Amplitude"=0.0, "omega(0)"=0.0, "Gamma"=0.0, "phase"=0.0, "Q"=0.0, "Norm  Ampl"=0.0, "z (inf)"=0.0+0.0i, "4corners"={"z (-pi/2)"=0.0+0.0i, "z(inf)"=0.0+0.0i, "z (pi/2)"=0.0+0.0i, "z center"=0.0+0.0i, "z(0)"=0.0+0.0i, "radius"=0.0}}, "timestamp(min)"=1965.933333337307, "timestamp"=timestamp(3493845777 s since 1904-01-01), "Magn Field(T)"=0.0}, {"temperature"=15.723, "lorentzian"={"Amplitude"=0.0, "omega(0)"=0.0, "Gamma"=0.0, "phase"=0.0, "Q"=0.0, "Norm  Ampl"=0.0, "z (inf)"=0.0+0.0i, "4corners"={"z (-pi/2)"=0.0+0.0i, "z(inf)"=0.0+0.0i, "z (pi/2)"=0.0+0.0i, "z center"=0.0+0.0i, "z(0)"=0.0+0.0i, "radius"=0.0}}, "timestamp(min)"=1967.25, "timestamp"=timestamp(3493845856 s since 1904-01-01), "Magn Field(T)"=0.0}, {"temperature"=15.622, "lorentzian"={"Amplitude"=0.0, "omega(0)"=0.0, "Gamma"=0.0, "phase"=0.0, "Q"=0.0, "Norm  Ampl"=0.0, "z (inf)"=0.0+0.0i, "4corners"={"z (-pi/2)"=0.0+0.0i, "z(inf)"=0.0+0.0i, "z (pi/2)"=0.0+0.0i, "z center"=0.0+0.0i, "z(0)"=0.0+0.0i, "radius"=0.0}}, "timestamp(min)"=1968.5833333358169, "timestamp"=timestamp(3493845936 s since 1904-01-01), "Magn Field(T)"=0.0}, {"temperature"=15.52, "lorentzian"={"Amplitude"=0.0, "omega(0)"=0.0, "Gamma"=0.0, "phase"=0.0, "Q"=0.0, "Norm  Ampl"=0.0, "z (inf)"=0.0+0.0i, "4corners"={"z (-pi/2)"=0.0+0.0i, "z(inf)"=0.0+0.0i, "z (pi/2)"=0.0+0.0i, "z center"=0.0+0.0i, "z(0)"=0.0+0.0i, "radius"=0.0}}, "timestamp(min)"=1969.8999999985099, "timestamp"=timestamp(3493846015 s since 1904-01-01), "Magn Field(T)"=0.0}, {"temperature"=15.419, "lorentzian"={"Amplitude"=0.0, "omega(0)"=0.0, "Gamma"=0.0, "phase"=0.0, "Q"=0.0, "Norm  Ampl"=0.0, "z (inf)"=0.0+0.0i, "4corners"={"z (-pi/2)"=0.0+0.0i, "z(inf)"=0.0+0.0i, "z (pi/2)"=0.0+0.0i, "z center"=0.0+0.0i, "z(0)"=0.0+0.0i, "radius"=0.0}}, "timestamp(min)"=1971.2333333343267, "timestamp"=timestamp(3493846095 s since 1904-01-01), "Magn Field(T)"=0.0}, {"temperature"=15.33, "lorentzian"={"Amplitude"=0.0, "omega(0)"=0.0, "Gamma"=0.0, "phase"=0.0, "Q"=0.0, "Norm  Ampl"=0.0, "z (inf)"=0.0+0.0i, "4corners"={"z (-pi/2)"=0.0+0.0i, "z(inf)"=0.0+0.0i, "z (pi/2)"=0.0+0.0i, "z center"=0.0+0.0i, "z(0)"=0.0+0.0i, "radius"=0.0}}, "timestamp(min)"=1972.5500000044703, "timestamp"=timestamp(3493846174 s since 1904-01-01), "Magn Field(T)"=0.0}, {"temperature"=15.223, "lorentzian"={"Amplitude"=0.0, "omega(0)"=0.0, "Gamma"=0.0, "phase"=0.0, "Q"=0.0, "Norm  Ampl"=0.0, "z (inf)"=0.0+0.0i, "4corners"={"z (-pi/2)"=0.0+0.0i, "z(inf)"=0.0+0.0i, "z (pi/2)"=0.0+0.0i, "z center"=0.0+0.0i, "z(0)"=0.0+0.0i, "radius"=0.0}}, "timestamp(min)"=1973.8666666671634, "timestamp"=timestamp(3493846253 s since 1904-01-01), "Magn Field(T)"=0.0}, {"temperature"=15.166, "lorentzian"={"Amplitude"=0.0, "omega(0)"=0.0, "Gamma"=0.0, "phase"=0.0, "Q"=0.0, "Norm  Ampl"=0.0, "z (inf)"=0.0+0.0i, "4corners"={"z (-pi/2)"=0.0+0.0i, "z(inf)"=0.0+0.0i, "z (pi/2)"=0.0+0.0i, "z center"=0.0+0.0i, "z(0)"=0.0+0.0i, "radius"=0.0}}, "timestamp(min)"=1975.2000000029802, "timestamp"=timestamp(3493846333 s since 1904-01-01), "Magn Field(T)"=0.0}, {"temperature"=15.139, "lorentzian"={"Amplitude"=0.0, "omega(0)"=0.0, "Gamma"=0.0, "phase"=0.0, "Q"=0.0, "Norm  Ampl"=0.0, "z (inf)"=0.0+0.0i, "4corners"={"z (-pi/2)"=0.0+0.0i, "z(inf)"=0.0+0.0i, "z (pi/2)"=0.0+0.0i, "z center"=0.0+0.0i, "z(0)"=0.0+0.0i, "radius"=0.0}}, "timestamp(min)"=1976.5166666656733, "timestamp"=timestamp(3493846412 s since 1904-01-01), "Magn Field(T)"=0.0}, {"temperature"=15.12, "lorentzian"={"Amplitude"=0.0, "omega(0)"=0.0, "Gamma"=0.0, "phase"=0.0, "Q"=0.0, "Norm  Ampl"=0.0, "z (inf)"=0.0+0.0i, "4corners"={"z (-pi/2)"=0.0+0.0i, "z(inf)"=0.0+0.0i, "z (pi/2)"=0.0+0.0i, "z center"=0.0+0.0i, "z(0)"=0.0+0.0i, "radius"=0.0}}, "timestamp(min)"=1977.8500000014901, "timestamp"=timestamp(3493846492 s since 1904-01-01), "Magn Field(T)"=0.0}, {"temperature"=15.102, "lorentzian"={"Amplitude"=0.0, "omega(0)"=0.0, "Gamma"=0.0, "phase"=0.0, "Q"=0.0, "Norm  Ampl"=0.0, "z (inf)"=0.0+0.0i, "4corners"={"z (-pi/2)"=0.0+0.0i, "z(inf)"=0.0+0.0i, "z (pi/2)"=0.0+0.0i, "z center"=0.0+0.0i, "z(0)"=0.0+0.0i, "radius"=0.0}}, "timestamp(min)"=1979.1666666641831, "timestamp"=timestamp(3493846571 s since 1904-01-01), "Magn Field(T)"=0.0}, {"temperature"=15.094, "lorentzian"={"Amplitude"=0.0, "omega(0)"=0.0, "Gamma"=0.0, "phase"=0.0, "Q"=0.0, "Norm  Ampl"=0.0, "z (inf)"=0.0+0.0i, "4corners"={"z (-pi/2)"=0.0+0.0i, "z(inf)"=0.0+0.0i, "z (pi/2)"=0.0+0.0i, "z center"=0.0+0.0i, "z(0)"=0.0+0.0i, "radius"=0.0}}, "timestamp(min)"=1980.4833333343267, "timestamp"=timestamp(3493846650 s since 1904-01-01), "Magn Field(T)"=0.0}, {"temperature"=15.075, "lorentzian"={"Amplitude"=0.0, "omega(0)"=0.0, "Gamma"=0.0, "phase"=0.0, "Q"=0.0, "Norm  Ampl"=0.0, "z (inf)"=0.0+0.0i, "4corners"={"z (-pi/2)"=0.0+0.0i, "z(inf)"=0.0+0.0i, "z (pi/2)"=0.0+0.0i, "z center"=0.0+0.0i, "z(0)"=0.0+0.0i, "radius"=0.0}}, "timestamp(min)"=1981.8166666701436, "timestamp"=timestamp(3493846730 s since 1904-01-01), "Magn Field(T)"=0.0}, {"temperature"=15.065, "lorentzian"={"Amplitude"=0.0, "omega(0)"=0.0, "Gamma"=0.0, "phase"=0.0, "Q"=0.0, "Norm  Ampl"=0.0, "z (inf)"=0.0+0.0i, "4corners"={"z (-pi/2)"=0.0+0.0i, "z(inf)"=0.0+0.0i, "z (pi/2)"=0.0+0.0i, "z center"=0.0+0.0i, "z(0)"=0.0+0.0i, "radius"=0.0}}, "timestamp(min)"=1983.1333333328366, "timestamp"=timestamp(3493846809 s since 1904-01-01), "Magn Field(T)"=0.0}, {"temperature"=15.054, "lorentzian"={"Amplitude"=0.0, "omega(0)"=0.0, "Gamma"=0.0, "phase"=0.0, "Q"=0.0, "Norm  Ampl"=0.0, "z (inf)"=0.0+0.0i, "4corners"={"z (-pi/2)"=0.0+0.0i, "z(inf)"=0.0+0.0i, "z (pi/2)"=0.0+0.0i, "z center"=0.0+0.0i, "z(0)"=0.0+0.0i, "radius"=0.0}}, "timestamp(min)"=1984.4500000029802, "timestamp"=timestamp(3493846888 s since 1904-01-01), "Magn Field(T)"=0.0}, {"temperature"=15.042, "lorentzian"={"Amplitude"=0.0, "omega(0)"=0.0, "Gamma"=0.0, "phase"=0.0, "Q"=0.0, "Norm  Ampl"=0.0, "z (inf)"=0.0+0.0i, "4corners"={"z (-pi/2)"=0.0+0.0i, "z(inf)"=0.0+0.0i, "z (pi/2)"=0.0+0.0i, "z center"=0.0+0.0i, "z(0)"=0.0+0.0i, "radius"=0.0}}, "timestamp(min)"=1985.7833333313465, "timestamp"=timestamp(3493846968 s since 1904-01-01), "Magn Field(T)"=0.0}, {"temperature"=15.031, "lorentzian"={"Amplitude"=0.0, "omega(0)"=0.0, "Gamma"=0.0, "phase"=0.0, "Q"=0.0, "Norm  Ampl"=0.0, "z (inf)"=0.0+0.0i, "4corners"={"z (-pi/2)"=0.0+0.0i, "z(inf)"=0.0+0.0i, "z (pi/2)"=0.0+0.0i, "z center"=0.0+0.0i, "z(0)"=0.0+0.0i, "radius"=0.0}}, "timestamp(min)"=1987.1000000014901, "timestamp"=timestamp(3493847047 s since 1904-01-01), "Magn Field(T)"=0.0}, {"temperature"=15.023, "lorentzian"={"Amplitude"=0.0, "omega(0)"=0.0, "Gamma"=0.0, "phase"=0.0, "Q"=0.0, "Norm  Ampl"=0.0, "z (inf)"=0.0+0.0i, "4corners"={"z (-pi/2)"=0.0+0.0i, "z(inf)"=0.0+0.0i, "z (pi/2)"=0.0+0.0i, "z center"=0.0+0.0i, "z(0)"=0.0+0.0i, "radius"=0.0}}, "timestamp(min)"=1988.433333337307, "timestamp"=timestamp(3493847127 s since 1904-01-01), "Magn Field(T)"=0.0}, {"temperature"=15.011, "lorentzian"={"Amplitude"=0.0, "omega(0)"=0.0, "Gamma"=0.0, "phase"=0.0, "Q"=0.0, "Norm  Ampl"=0.0, "z (inf)"=0.0+0.0i, "4corners"={"z (-pi/2)"=0.0+0.0i, "z(inf)"=0.0+0.0i, "z (pi/2)"=0.0+0.0i, "z center"=0.0+0.0i, "z(0)"=0.0+0.0i, "radius"=0.0}}, "timestamp(min)"=1989.75, "timestamp"=timestamp(3493847206 s since 1904-01-01), "Magn Field(T)"=0.0}, {"temperature"=15.012, "lorentzian"={"Amplitude"=0.0, "omega(0)"=0.0, "Gamma"=0.0, "phase"=0.0, "Q"=0.0, "Norm  Ampl"=0.0, "z (inf)"=0.0+0.0i, "4corners"={"z (-pi/2)"=0.0+0.0i, "z(inf)"=0.0+0.0i, "z (pi/2)"=0.0+0.0i, "z center"=0.0+0.0i, "z(0)"=0.0+0.0i, "radius"=0.0}}, "timestamp(min)"=1991.0666666701436, "timestamp"=timestamp(3493847285 s since 1904-01-01), "Magn Field(T)"=0.0}, {"temperature"=15.016, "lorentzian"={"Amplitude"=0.0, "omega(0)"=0.0, "Gamma"=0.0, "phase"=0.0, "Q"=0.0, "Norm  Ampl"=0.0, "z (inf)"=0.0+0.0i, "4corners"={"z (-pi/2)"=0.0+0.0i, "z(inf)"=0.0+0.0i, "z (pi/2)"=0.0+0.0i, "z center"=0.0+0.0i, "z(0)"=0.0+0.0i, "radius"=0.0}}, "timestamp(min)"=1992.3999999985099, "timestamp"=timestamp(3493847365 s since 1904-01-01), "Magn Field(T)"=0.0}, {"temperature"=15.007, "lorentzian"={"Amplitude"=0.0, "omega(0)"=0.0, "Gamma"=0.0, "phase"=0.0, "Q"=0.0, "Norm  Ampl"=0.0, "z (inf)"=0.0+0.0i, "4corners"={"z (-pi/2)"=0.0+0.0i, "z(inf)"=0.0+0.0i, "z (pi/2)"=0.0+0.0i, "z center"=0.0+0.0i, "z(0)"=0.0+0.0i, "radius"=0.0}}, "timestamp(min)"=1993.7166666686535, "timestamp"=timestamp(3493847444 s since 1904-01-01), "Magn Field(T)"=0.0}, {"temperature"=15.003, "lorentzian"={"Amplitude"=0.0, "omega(0)"=0.0, "Gamma"=0.0, "phase"=0.0, "Q"=0.0, "Norm  Ampl"=0.0, "z (inf)"=0.0+0.0i, "4corners"={"z (-pi/2)"=0.0+0.0i, "z(inf)"=0.0+0.0i, "z (pi/2)"=0.0+0.0i, "z center"=0.0+0.0i, "z(0)"=0.0+0.0i, "radius"=0.0}}, "timestamp(min)"=1995.0333333313465, "timestamp"=timestamp(3493847523 s since 1904-01-01), "Magn Field(T)"=0.0}, {"temperature"=14.997, "lorentzian"={"Amplitude"=0.0, "omega(0)"=0.0, "Gamma"=0.0, "phase"=0.0, "Q"=0.0, "Norm  Ampl"=0.0, "z (inf)"=0.0+0.0i, "4corners"={"z (-pi/2)"=0.0+0.0i, "z(inf)"=0.0+0.0i, "z (pi/2)"=0.0+0.0i, "z center"=0.0+0.0i, "z(0)"=0.0+0.0i, "radius"=0.0}}, "timestamp(min)"=1996.3666666671634, "timestamp"=timestamp(3493847603 s since 1904-01-01), "Magn Field(T)"=0.0}, {"temperature"=14.985, "lorentzian"={"Amplitude"=0.0, "omega(0)"=0.0, "Gamma"=0.0, "phase"=0.0, "Q"=0.0, "Norm  Ampl"=0.0, "z (inf)"=0.0+0.0i, "4corners"={"z (-pi/2)"=0.0+0.0i, "z(inf)"=0.0+0.0i, "z (pi/2)"=0.0+0.0i, "z center"=0.0+0.0i, "z(0)"=0.0+0.0i, "radius"=0.0}}, "timestamp(min)"=1997.683333337307, "timestamp"=timestamp(3493847682 s since 1904-01-01), "Magn Field(T)"=0.0}, {"temperature"=14.981, "lorentzian"={"Amplitude"=0.0, "omega(0)"=0.0, "Gamma"=0.0, "phase"=0.0, "Q"=0.0, "Norm  Ampl"=0.0, "z (inf)"=0.0+0.0i, "4corners"={"z (-pi/2)"=0.0+0.0i, "z(inf)"=0.0+0.0i, "z (pi/2)"=0.0+0.0i, "z center"=0.0+0.0i, "z(0)"=0.0+0.0i, "radius"=0.0}}, "timestamp(min)"=1999.0166666656733, "timestamp"=timestamp(3493847762 s since 1904-01-01), "Magn Field(T)"=0.0}, {"temperature"=14.976, "lorentzian"={"Amplitude"=0.0, "omega(0)"=0.0, "Gamma"=0.0, "phase"=0.0, "Q"=0.0, "Norm  Ampl"=0.0, "z (inf)"=0.0+0.0i, "4corners"={"z (-pi/2)"=0.0+0.0i, "z(inf)"=0.0+0.0i, "z (pi/2)"=0.0+0.0i, "z center"=0.0+0.0i, "z(0)"=0.0+0.0i, "radius"=0.0}}, "timestamp(min)"=2000.3333333358169, "timestamp"=timestamp(3493847841 s since 1904-01-01), "Magn Field(T)"=0.0}, {"temperature"=14.967, "lorentzian"={"Amplitude"=0.0, "omega(0)"=0.0, "Gamma"=0.0, "phase"=0.0, "Q"=0.0, "Norm  Ampl"=0.0, "z (inf)"=0.0+0.0i, "4corners"={"z (-pi/2)"=0.0+0.0i, "z(inf)"=0.0+0.0i, "z (pi/2)"=0.0+0.0i, "z center"=0.0+0.0i, "z(0)"=0.0+0.0i, "radius"=0.0}}, "timestamp(min)"=2001.6499999985099, "timestamp"=timestamp(3493847920 s since 1904-01-01), "Magn Field(T)"=0.0}, {"temperature"=14.967, "lorentzian"={"Amplitude"=0.0, 
